vi "Regular Timer Action Engine.vi"(0 "Enum":T1, 1 "Time Target":dbl, 3 "error in":errorcluster) -> (7 "Status":cluster{"Running":bool, "Done":bool}, 10 "error out":errorcluster)   [LabVIEW 2014]
uses:
  Control Timer.ctl
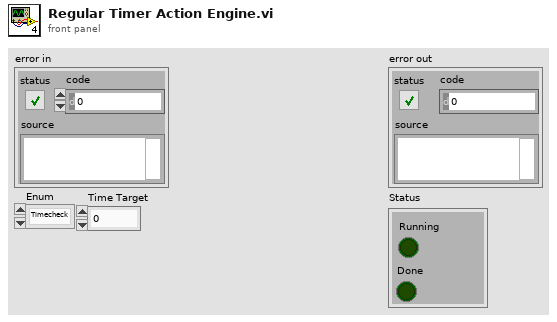
[diagram p1: front panel]
types:
  T1 = typedef "Control Timer.ctl" = enum16{"Timecheck", "Reset"}
  T2 = cluster{"Last Time Stamp":dbl, "Elapsed Time":dbl}
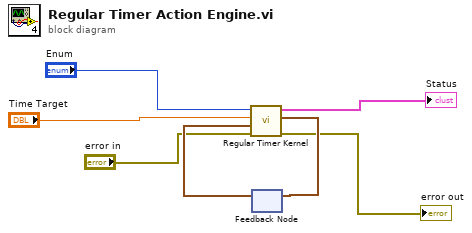
[diagram p0: block diagram]
diagram:
  n1 = feedback #1() -> (w6:T2)  [unwired: 1 in]
  n2 = call "Regular Timer Kernel.vi"("error in"="error in", "Timer Data In"=w6, "Time Target"="Time Target", "Enum"="Enum") -> ("error out"=→"error out":errorcluster, "Timer Data Out"=w7:T2, "Status"=→"Status":cluster{"Running":bool, "Done":bool})  [unwired: 5 in]
  n3 = feedback-in #1(w7) -> ()
